vi "Controller.vi"(8 "Error In":errorcluster) -> (0 "Error Out":errorcluster)   [LabVIEW 2017]
uses:
  Controller Data Cluster.ctl
  User Console/UI Data Cluster.ctl
  Timed Action.ctl
  Current Direction.ctl
  Communication/Reference Action.ctl
  Display Console/Communication/Display Console Message.ctl
  Display Console/Display Console Data Cluster.ctl
  Communication/User Event/User Event Cluster.ctl
  Communication/User Event/User Event Enum.ctl
  Communication/Controller Queue Message.ctl
  Support VIs/Timer Actions.ctl
  Emergency Enum.ctl
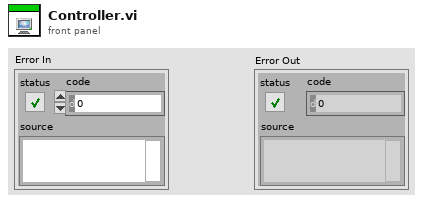
[diagram p1: front panel]
types:
  T1 = typedef "Controller Data Cluster.ctl" = cluster{"UI Data Cluster":T2, "Sensor Position":u32, "Module Closed?":cluster{"Display Loop":bool, "Sensor Loop ":bool}, "Time to Elapse":u32, "Request?":bool, "Timed Action":T3, "Time Constants":cluster{"Open Door":dbl, "Close Door":dbl, "Travel":dbl, "Inactivity":dbl}, "Inactivity":bool, "Current Floor":u32, "Current Direction":T4, "Travel?":bool, "Program Exit":bool[], "Emergency?":bool}
  T2 = typedef "UI Data Cluster.ctl" = cluster{"Floor Selection":bool[], "Elevator Call Up":bool[], "Elevator Call Down":bool[], "Door Buttons":cluster{"Open":bool, "Close":bool}, "Emergency":bool}
  T3 = typedef "Timed Action.ctl" = enum16{"Open Door", "Close Door", "Travel", "Inactivity"}
  T4 = typedef "Current Direction.ctl" = enum16{"Up", "Down", "Idle"}
  T5 = typedef "Reference Action.ctl" = enum16{"Set", "Get"}
  T6 = typedef "Controller Queue Message.ctl" = enum16{"Initialize", "User Console Update", "Sensor Update", "Wait for First Request", "Start and Move", "Analysis", "Continue Travel", "Stop at Floor", "Open and Close Door Sequence", "Close Door", "No Request Remaining", "Check Time", "Emergency Call", "Terminate Process", "Controller Exit", "Start Exit", "Error Handling"}
  T7 = typedef "Display Console Message.ctl" = enum16{"Update Location", "Initialize", "Update", "Update Time", "Update Emergency", "Errror Handling", "Exit"}
  T8 = typedef "Timer Actions.ctl" = enum16{"Reset", "Check Time"}
  T9 = typedef "Display Console Data Cluster.ctl" = cluster{"Timing":dbl, "Elevator Location":u32, "Elevator Direction":cluster{"Up":bool, "Down":bool}, "Door Open":bool, "Emergency":bool}
  T10 = typedef "User Event Enum.ctl" = enum16{"Update Controlls", "Disable Open/Close Controlls", "Disable Open Door Controll", "Enable Open/Close Controlls", "Disable All Controlls", "Controller Loop Closed"}
  T11 = typedef "Emergency Enum.ctl" = enum16{"Energency On", "Emergency Off", "Emergency Idle"}
  T12 = typedef "User Event Cluster.ctl" = cluster{"User Event Enum":T10, "UI Data Cluster":T2}
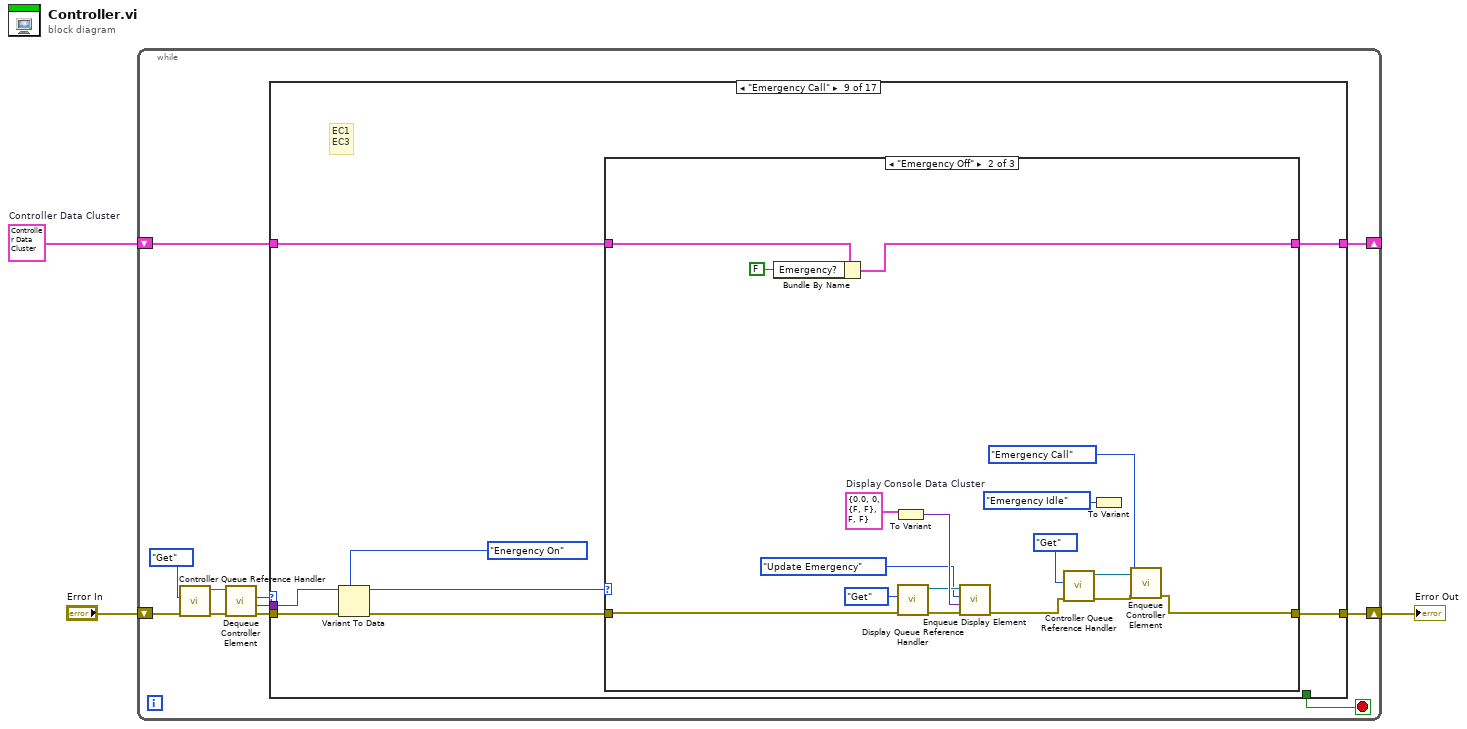
[diagram p0: block diagram]
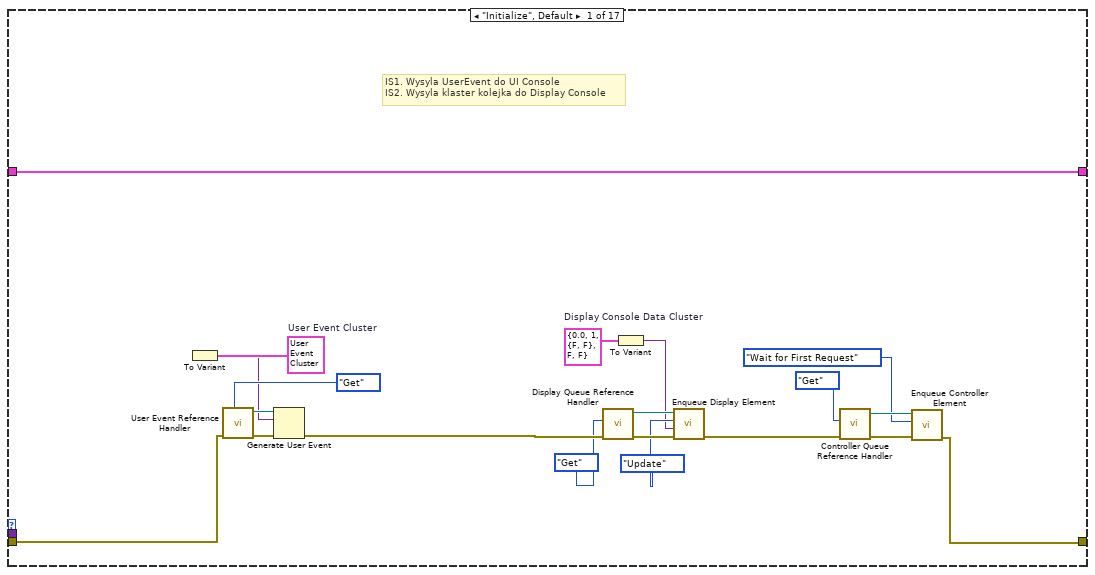
[diagram p2: hidden frame]
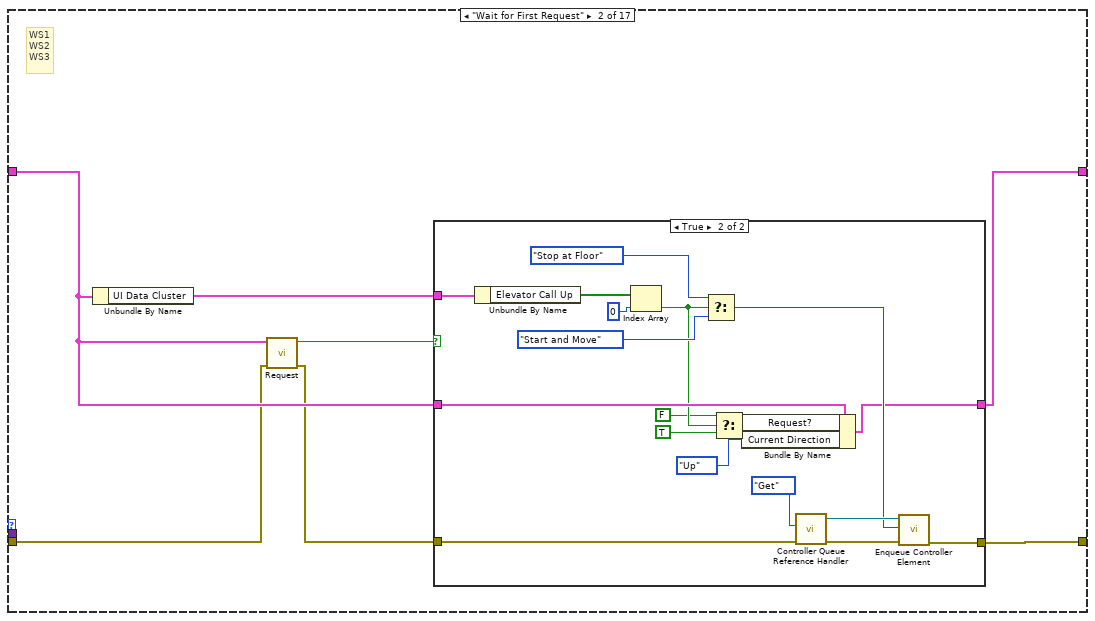
[diagram p3: hidden frame]
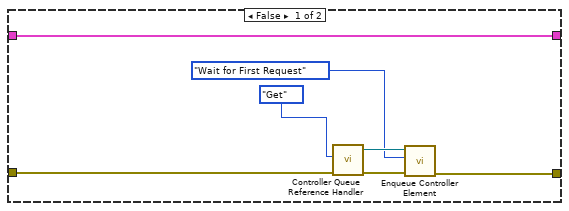
[diagram p4: hidden frame]
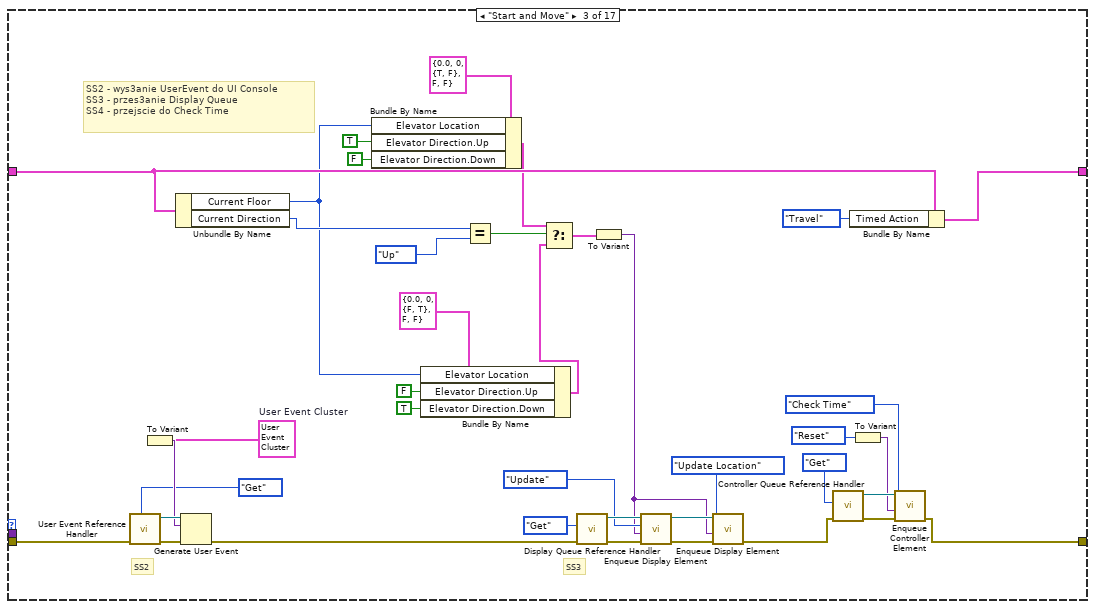
[diagram p5: hidden frame]
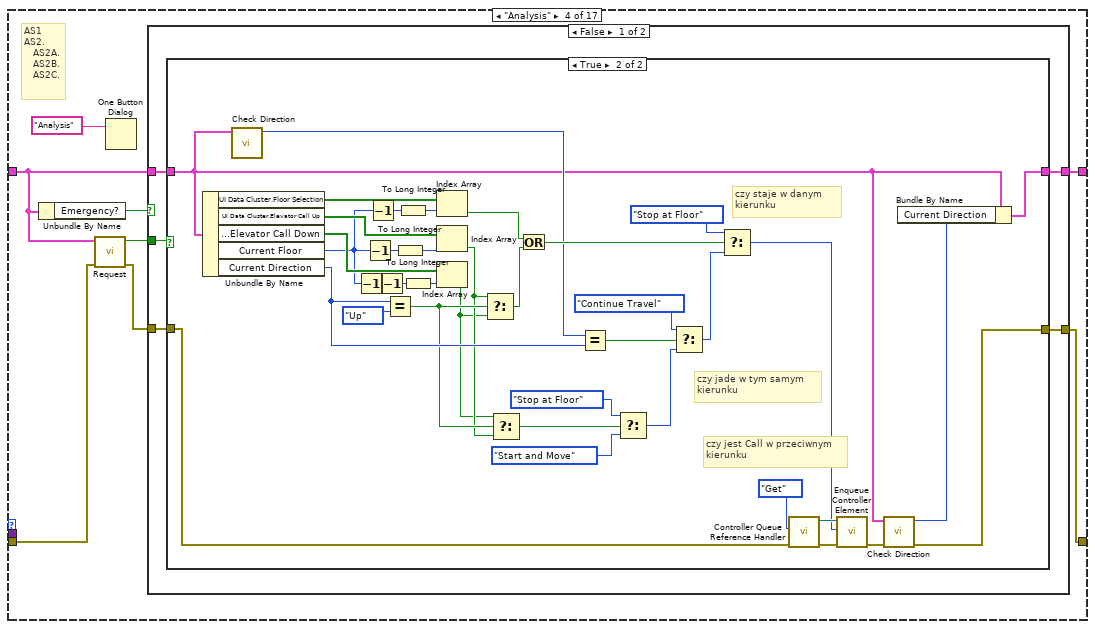
[diagram p6: hidden frame]
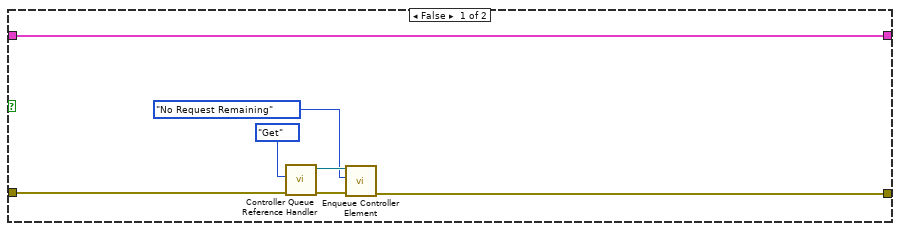
[diagram p7: hidden frame]
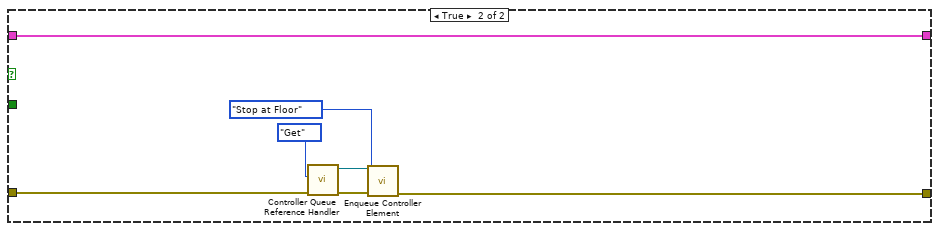
[diagram p8: hidden frame]
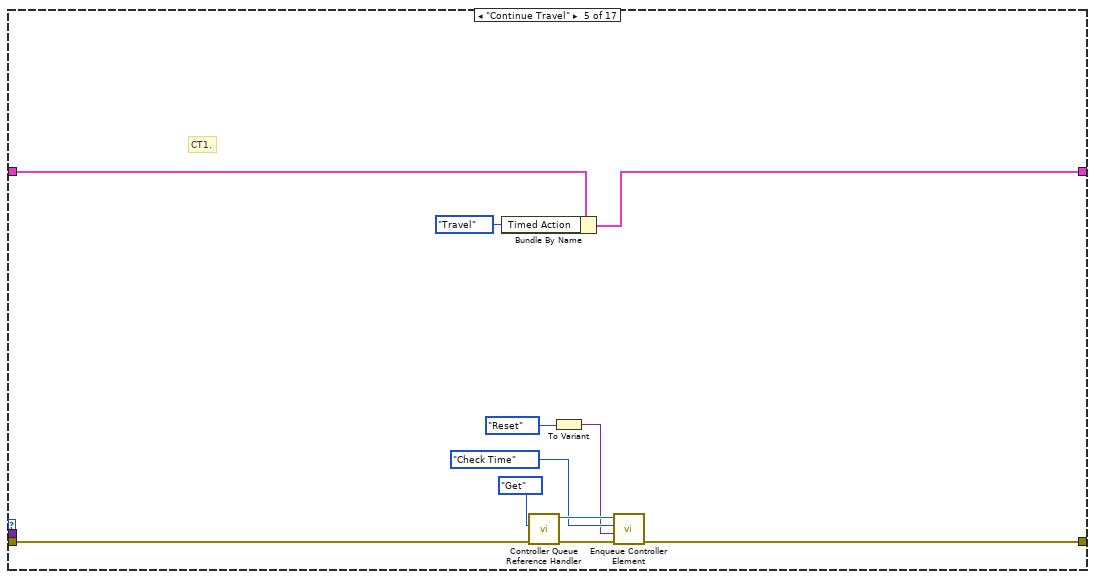
[diagram p9: hidden frame]
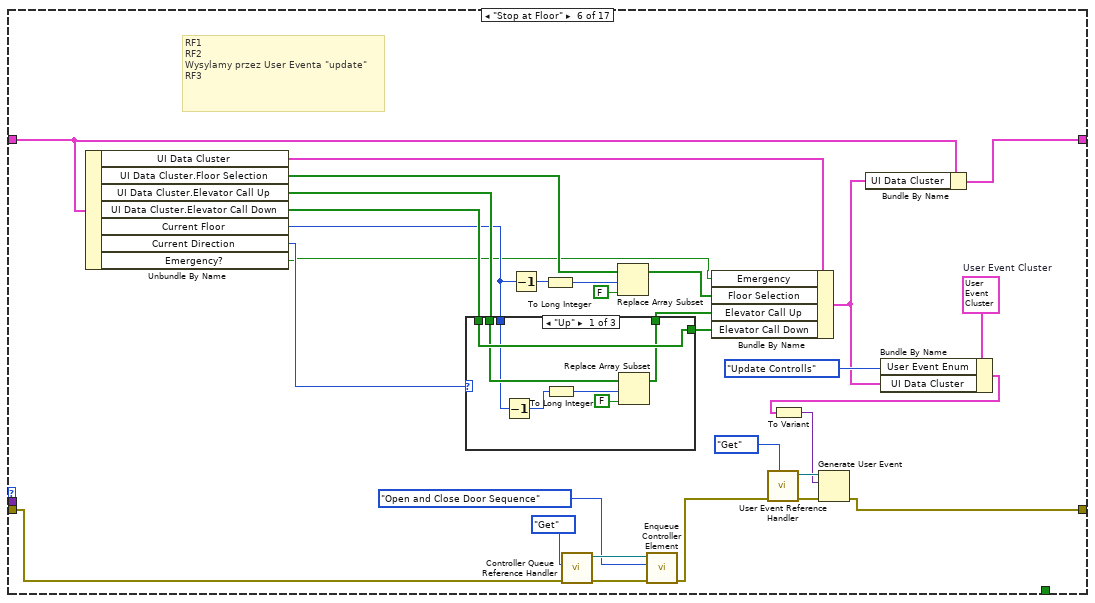
[diagram p10: hidden frame]
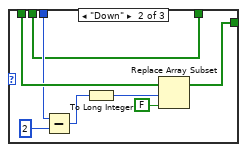
[diagram p11: hidden frame]
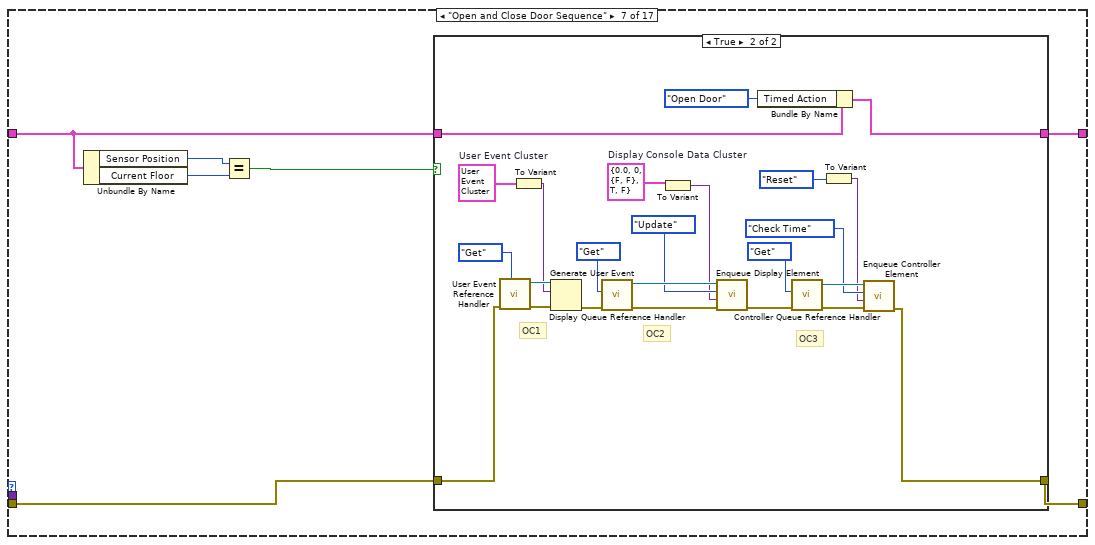
[diagram p13: hidden frame]
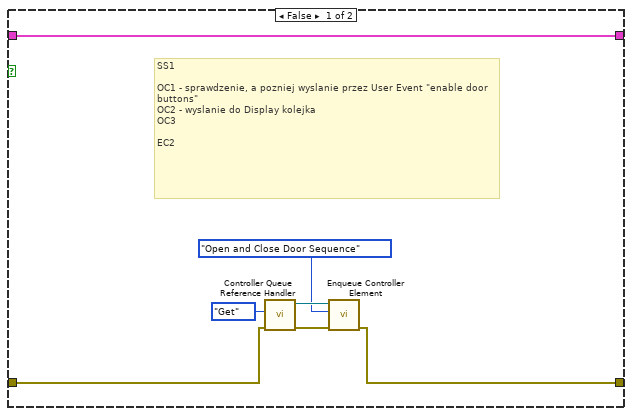
[diagram p14: hidden frame]
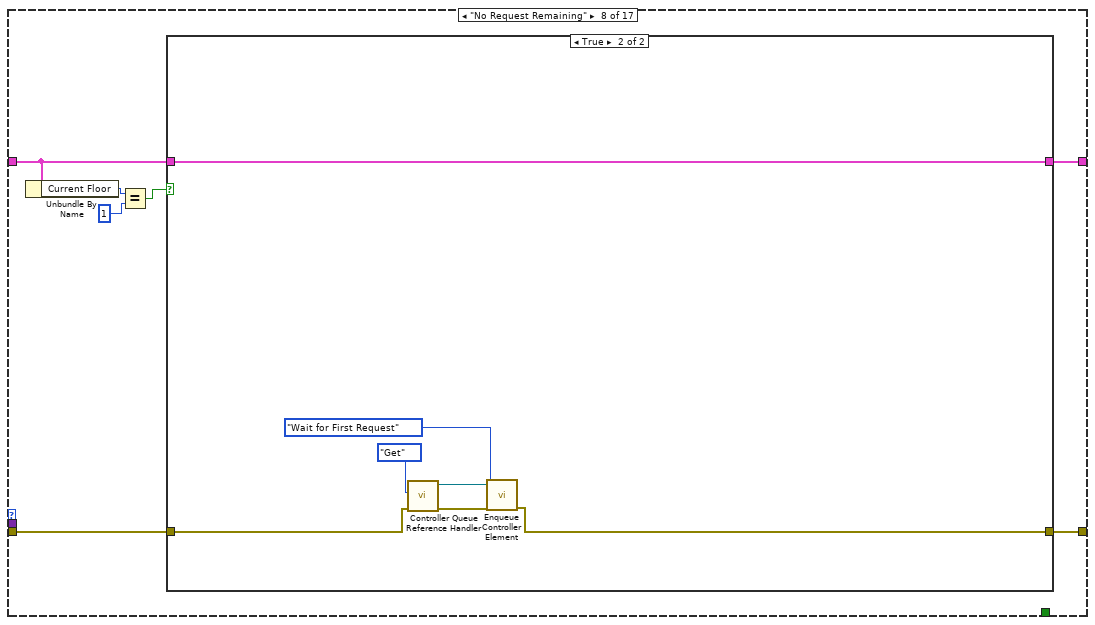
[diagram p15: hidden frame]
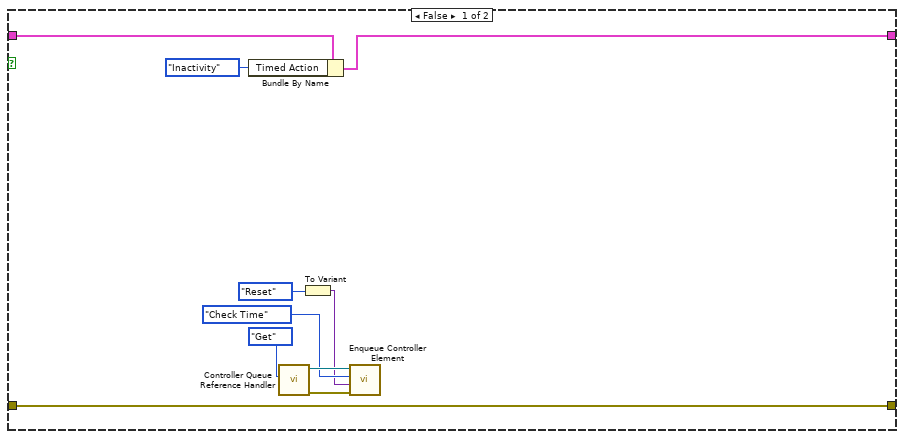
[diagram p16: hidden frame]
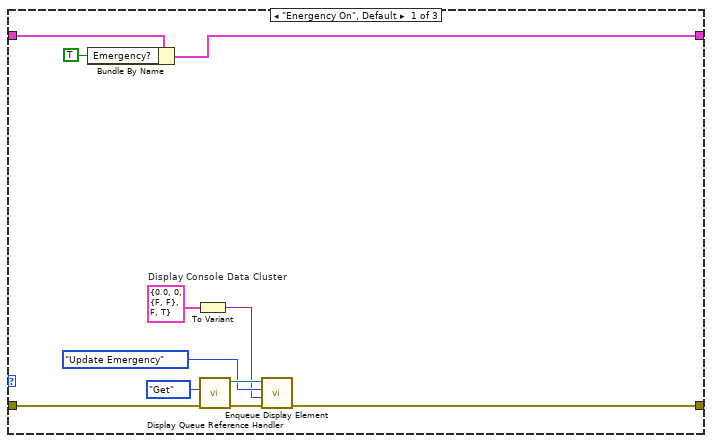
[diagram p17: hidden frame]
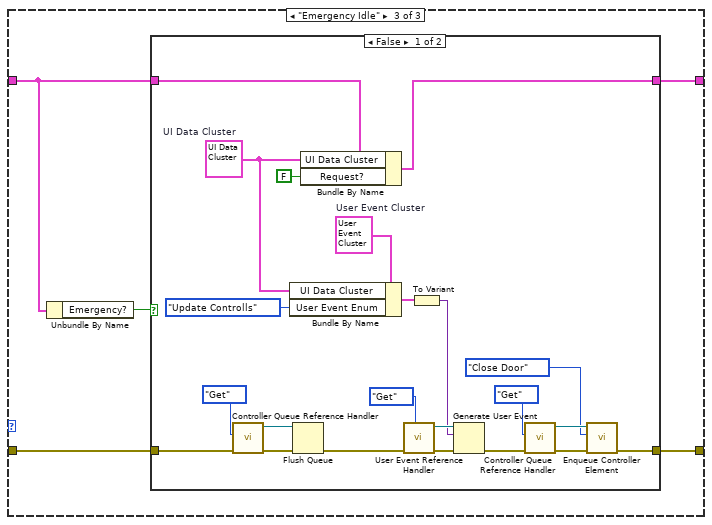
[diagram p18: hidden frame]
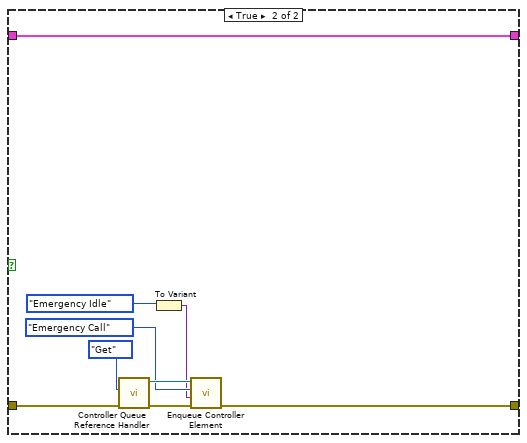
[diagram p19: hidden frame]
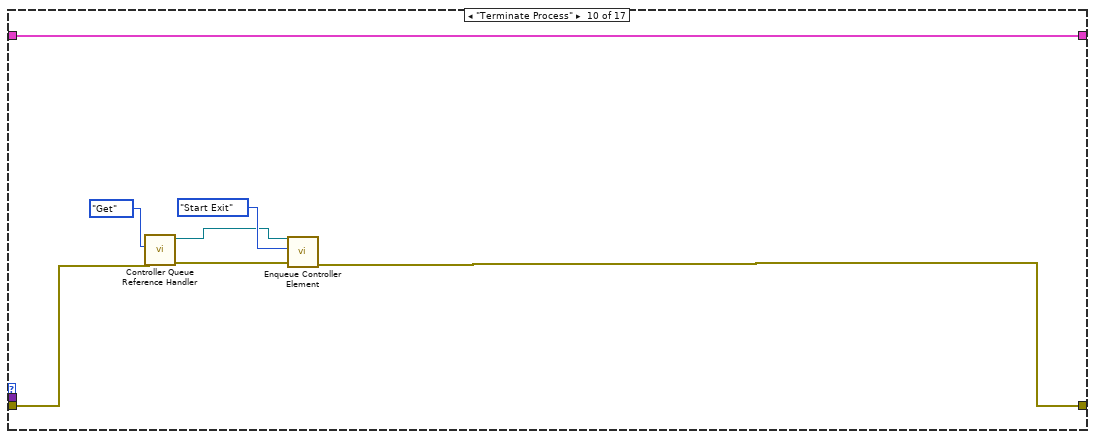
[diagram p20: hidden frame]
diagram:
  w1 = T1 {"UI Data Cluster"={"Floor Selection"=[], "Elevator Call Up"=[], "Elevator Call Down"=[], "Door Buttons"={"Open"=FALSE, "Close"=FALSE}, "Emergency"=FALSE}, "Sensor Position"=1, "Module Closed?"={"Display Loop"=FALSE, "Sensor Loop "=FALSE}, "Time to Elapse"=0, "Request?"=FALSE, "Timed Action"=enum."Open Door", "Time Constants"={"Open Door"=5.0, "Close Door"=1.0, "Travel"=10.0, "Inactivity"=20.0}, "Inactivity"=FALSE, "Current Floor"=1, "Current Direction"=enum."Idle", "Travel?"=FALSE, "Program Exit"=[], "Emergency?"=FALSE}  # Controller Data Cluster
  n1 = while {
    shift-right: [w12] -> w2
    shift-left: "Error In" -> [w14]
    shift-right: [w4] -> _
    shift-left: w1 -> [w7]
    stop <- w6 stop-if-true
    n2 = call "Controller Queue Reference Handler.vi"("Error In"=w14, "Reference Action"=Reference_Action."Get") -> ("Error Out"=w11:errorcluster, "Queue Ref Out"=w10:refnum<queue>)  [unwired: 8 in]
    n3 = call "Dequeue Controller Element.vi"("error in (no error)"=w11, "Message Queue"=w10) -> ("error out"=w8:errorcluster, "Controller Queue Data"=w5:variant, "Controller Queue Message"=w9:T6)  [unwired: 6 in, 1 out]
    n4 = case shown="\"Emergency Call\"" w9 {
      tunnel: w8 -> [w24 w37 w100 w107 w172 w185 w232 w269 w298 w365 w382 w388 w399 w405 w414 w659 w697]
      tunnel: [w15 w40 w84 w113 w171 w183 w231 w270 w293 w363 w381 w388 w398 w405 w408 w666 w678] -> w12
      tunnel: w7 -> [w32 w38 w89 w109 w180 w190 w230 w267 w291 w369 w371 w387 w392 w402 w410 w677 w693]
      tunnel: [w32 w39 w88 w112 w179 w195 w229 w268 w292 w369 w370 w387 w391 w401 w411 w677 w692] -> w4
      tunnel: [_ _ _ _ _ _ _ _ _ _ w374 _ _ _ _ _ _] -> w6
      tunnel: w5 -> [_ _ _ _ _ _ _ _ w297 _ w386 _ w400 w406 w415 _ _]
      frame "Initialize", Default {
        w22 = T12 {"User Event Enum"=enum."Update Controlls", "UI Data Cluster"={"Floor Selection"=[FALSE, FALSE, FALSE, FALSE], "Elevator Call Up"=[FALSE, FALSE, FALSE], "Elevator Call Down"=[FALSE, FALSE, FALSE], "Door Buttons"={"Open"=FALSE, "Close"=FALSE}, "Emergency"=FALSE}}  # User Event Cluster
        w25 = T9 {"Timing"=0.0, "Elevator Location"=1, "Elevator Direction"={"Up"=FALSE, "Down"=FALSE}, "Door Open"=FALSE, "Emergency"=FALSE}  # Display Console Data Cluster
        # "IS1. Wysyla UserEvent do UI Console \nIS2. Wysyla klaster kolejka do Display Console"
        n5 = To Variant(anything=w22) -> (Variant=w21:variant)
        n6 = call "User Event Reference Handler.vi"("Reference Action"=Reference_Action."Get", "Error In"=w24) -> ("Error Out"=w33:errorcluster, "User Event Refnum Out"=w34:refnum<user-event>)  [unwired: 7 in, 1 out]
        n7 = Generate User Event(user event=w34, event data cluster=w21, error in=w33) -> (error out=w29:errorcluster)  [unwired: 1 in, 1 out]
        n8 = call "Display Queue Reference Handler.vi"("Error In"=w29, "Reference Action"=Reference_Action."Get") -> ("Error Out"=w30:errorcluster, "Queue Ref Out"=w31:refnum<queue>)  [unwired: 8 in]
        n9 = To Variant(anything=w25) -> (Variant=w26:variant)
        n10 = call "Enqueue Display Element.vi"("error in (no error)"=w30, "Display Console Data"=w26, "Display Console Message"=Display_Console_Message."Update", "Message Queue"=w31) -> ("error out"=w16:errorcluster)  [unwired: 6 in, 1 out]
        n11 = call "Controller Queue Reference Handler.vi"("Error In"=w16, "Reference Action"=Reference_Action."Get") -> ("Error Out"=w19:errorcluster, "Queue Ref Out"=w18:refnum<queue>)  [unwired: 8 in]
        n12 = call "Enqueue Controller Element.vi"("error in (no error)"=w19, "Controller Queue Message"=Controller_Queue_Message."Wait for First Request", "Message Queue"=w18) -> ("error out"=w15:errorcluster)  [unwired: 7 in, 1 out]
      }
      frame "Wait for First Request" {
        # "WS1\nWS2\nWS3"
        n13 = Unbundle By Name(w38) -> ("UI Data Cluster"=w41:T2)
        n14 = call "Request.vi"("error in (no error)"=w37, "Controller Data Cluster"=w38) -> ("error out"=w36:errorcluster, "Request?"=w35:bool)  [unwired: 8 in]
        n15 = case shown="True" w35 {
          tunnel: w41 -> [_ w66]
          tunnel: w36 -> [w44 w57]
          tunnel: [w43 w56] -> w40
          tunnel: w38 -> [w42 w55]
          tunnel: [w42 w50] -> w39
          frame False {
            n16 = call "Controller Queue Reference Handler.vi"("Error In"=w44, "Reference Action"=Reference_Action."Get") -> ("Error Out"=w47:errorcluster, "Queue Ref Out"=w46:refnum<queue>)  [unwired: 8 in]
            n17 = call "Enqueue Controller Element.vi"("error in (no error)"=w47, "Controller Queue Message"=Controller_Queue_Message."Wait for First Request", "Message Queue"=w46) -> ("error out"=w43:errorcluster)  [unwired: 7 in, 1 out]
          }
          frame True {
            n18 = Unbundle By Name(w66) -> ("Elevator Call Up"=w65:bool[])
            n19 = Index Array(array=w65, index=0) -> (element=w53:bool)
            n20 = Select(t=Controller_Queue_Message."Stop at Floor" ("Controller Queue Message"), s=w53, f=Controller_Queue_Message."Start and Move" ("Controller Queue Message")) -> (s? t:f=w58:T6)
            n21 = Select(t=FALSE, s=w53, f=TRUE) -> (s? t:f=w54:bool)
            n22 = Bundle By Name(cluster=w55, "Request?"=w54, "Current Direction"=Current_Direction."Up") -> (w50:T1)
            n23 = call "Controller Queue Reference Handler.vi"("Error In"=w57, "Reference Action"=Reference_Action."Get") -> ("Error Out"=w62:errorcluster, "Queue Ref Out"=w61:refnum<queue>)  [unwired: 8 in]
            n24 = call "Enqueue Controller Element.vi"("error in (no error)"=w62, "Controller Queue Message"=w58, "Message Queue"=w61) -> ("error out"=w56:errorcluster)  [unwired: 7 in, 1 out]
          }
        }
      }
      frame "Start and Move" {
        w101 = T12 {"User Event Enum"=enum."Disable Open/Close Controlls", "UI Data Cluster"={"Floor Selection"=[], "Elevator Call Up"=[], "Elevator Call Down"=[], "Door Buttons"={"Open"=FALSE, "Close"=FALSE}, "Emergency"=FALSE}}  # User Event Cluster
        # "SS3"
        # "SS2"
        # "SS2 - wys3anie UserEvent do UI Console\nSS3 - przes3anie Display Queue\nSS4 - przejscie do Check Time"
        n25 = call "User Event Reference Handler.vi"("Reference Action"=Reference_Action."Get", "Error In"=w100) -> ("Error Out"=w103:errorcluster, "User Event Refnum Out"=w105:refnum<user-event>)  [unwired: 7 in, 1 out]
        n26 = To Variant(anything=w101) -> (Variant=w104:variant)
        n27 = Unbundle By Name(w89) -> ("Current Floor"=w76:u32, "Current Direction"=w99:T4)
        n28 = Generate User Event(user event=w105, event data cluster=w104, error in=w103) -> (error out=w91:errorcluster)  [unwired: 1 in, 1 out]
        n29 = Bundle By Name(cluster=T9 {"Timing"=0.0, "Elevator Location"=0, "Elevator Direction"={"Up"=TRUE, "Down"=FALSE}, "Door Open"=FALSE, "Emergency"=FALSE} ("Display Console Data Cluster"), "Elevator Location"=w76, "Elevator Direction.Up"=TRUE, "Elevator Direction.Down"=FALSE) -> (w78:T9)
        n30 = Bundle By Name(cluster=T9 {"Timing"=0.0, "Elevator Location"=0, "Elevator Direction"={"Up"=FALSE, "Down"=TRUE}, "Door Open"=FALSE, "Emergency"=FALSE} ("Display Console Data Cluster"), "Elevator Location"=w76, "Elevator Direction.Up"=FALSE, "Elevator Direction.Down"=TRUE) -> (w72:T9)
        n31 = Equal?(x=w99, y=Current_Direction."Up" ("Current Direction")) -> (x = y?=w97:bool)
        n32 = Select(t=w78, s=w97, f=w72) -> (s? t:f=w92:T9)
        n33 = call "Display Queue Reference Handler.vi"("Error In"=w91, "Reference Action"=Reference_Action."Get") -> ("Error Out"=w95:errorcluster, "Queue Ref Out"=w94:refnum<queue>)  [unwired: 8 in]
        n34 = To Variant(anything=w92) -> (Variant=w67:variant)
        n35 = call "Enqueue Display Element.vi"("error in (no error)"=w95, "Display Console Data"=w67, "Display Console Message"=Display_Console_Message."Update", "Message Queue"=w94) -> ("error out"=w71:errorcluster, "dup Message Queue"=w69:refnum<queue>)  [unwired: 6 in]
        n36 = call "Enqueue Display Element.vi"("error in (no error)"=w71, "Display Console Data"=w67, "Display Console Message"=Display_Console_Message."Update Location", "Message Queue"=w69) -> ("error out"=w70:errorcluster)  [unwired: 6 in, 1 out]
        n37 = call "Controller Queue Reference Handler.vi"("Error In"=w70, "Reference Action"=Reference_Action."Get") -> ("Error Out"=w86:errorcluster, "Queue Ref Out"=w85:refnum<queue>)  [unwired: 8 in]
        n38 = Bundle By Name(cluster=w89, "Timed Action"=Timed_Action."Travel") -> (w88:T1)
        n39 = To Variant(anything=Timer_Actions."Reset" ("TimerAction")) -> (Variant=w81:variant)
        n40 = call "Enqueue Controller Element.vi"("error in (no error)"=w86, "Controller Queue Data"=w81, "Controller Queue Message"=Controller_Queue_Message."Check Time", "Message Queue"=w85) -> ("error out"=w84:errorcluster)  [unwired: 6 in, 1 out]
      }
      frame "Analysis" {
        # "AS1\nAS2.\n   AS2A.\n   AS2B.\n   AS2C."
        n41 = Unbundle By Name(w109) -> ("Emergency?"=w110:bool)
        n42 = call "Request.vi"("error in (no error)"=w107, "Controller Data Cluster"=w109) -> ("error out"=w106:errorcluster, "Request?"=w108:bool)  [unwired: 8 in]
        n43 = One Button Dialog(message="Analysis") -> ()  [unwired: 1 in, 1 out]
        n44 = case shown="False" w110 {
          tunnel: w106 -> [w117 w167]
          tunnel: [w116 w166] -> w113
          tunnel: [w114 w164] -> w112
          tunnel: w109 -> [w115 w164]
          tunnel: w108 -> [w118 _]
          frame False {
            n45 = case shown="True" w118 {
              tunnel: w117 -> [w121 w130]
              tunnel: [w120 w126] -> w116
              tunnel: w115 -> [w119 w128]
              tunnel: [w119 w147] -> w114
              frame False {
                n46 = call "Controller Queue Reference Handler.vi"("Error In"=w121, "Reference Action"=Reference_Action."Get") -> ("Error Out"=w124:errorcluster, "Queue Ref Out"=w125:refnum<queue>)  [unwired: 8 in]
                n47 = call "Enqueue Controller Element.vi"("error in (no error)"=w124, "Controller Queue Message"=Controller_Queue_Message."No Request Remaining", "Message Queue"=w125) -> ("error out"=w120:errorcluster)  [unwired: 7 in, 1 out]
              }
              frame True {
                # "czy jest Call w przeciwnym\nkierunku"
                # "czy jade w tym samym \nkierunku"
                # "czy staje w danym kierunku"
                n48 = Unbundle By Name(w128) -> ("UI Data Cluster.Floor Selection"=w162:bool[], "UI Data Cluster.Elevator Call Up"=w159:bool[], "UI Data Cluster.Elevator Call Down"=w156:bool[], "Current Floor"=w155:u32, "Current Direction"=w145:T4)
                n49 = call "Check Direction.vi"("Controller Data Cluster"=w128) -> ("Direction"=w146:T4)  [unwired: 9 in, 1 out]
                n50 = Decrement(x=w155) -> (x-1=w154:u32)
                n51 = Decrement(x=w155) -> (x-1=w158:u32)
                n52 = Decrement(x=w155) -> (x-1=w161:u32)
                n53 = Decrement(x=w154) -> (x-1=w153:u32)
                n54 = Equal?(x=w145, y=Current_Direction."Up") -> (x = y?=w141:bool)
                n55 = To Long Integer(number=w158) -> (32bit integer=w157:i32)
                n56 = To Long Integer(number=w161) -> (32bit integer=w160:i32)
                n57 = To Long Integer(number=w153) -> (32bit integer=w152:i32)
                n58 = Index Array(array=w162, index=w160) -> (element=w151:bool)
                n59 = Index Array(array=w159, index=w157) -> (element=w140:bool)
                n60 = Index Array(array=w156, index=w152) -> (element=w139:bool)
                n61 = Select(t=w140, s=w141, f=w139) -> (s? t:f=w150:bool)
                n62 = Select(t=w139, s=w141, f=w140) -> (s? t:f=w138:bool)
                n63 = Or(x=w151, y=w150) -> (x .or. y?=w149:bool)
                n64 = Equal?(x=w146, y=w145) -> (x = y?=w144:bool)
                n65 = Select(t=Controller_Queue_Message."Stop at Floor" ("Controller Queue Message"), s=w138, f=Controller_Queue_Message."Start and Move") -> (s? t:f=w135:T6)
                n66 = Select(t=Controller_Queue_Message."Continue Travel" ("Controller Queue Message"), s=w144, f=w135) -> (s? t:f=w142:T6)
                n67 = Select(t=Controller_Queue_Message."Stop at Floor" ("Controller Queue Message"), s=w149, f=w142) -> (s? t:f=w131:T6)
                n68 = call "Controller Queue Reference Handler.vi"("Error In"=w130, "Reference Action"=Reference_Action."Get") -> ("Error Out"=w133:errorcluster, "Queue Ref Out"=w132:refnum<queue>)  [unwired: 8 in]
                n69 = call "Enqueue Controller Element.vi"("error in (no error)"=w133, "Controller Queue Message"=w131, "Message Queue"=w132) -> ("error out"=w129:errorcluster)  [unwired: 7 in, 1 out]
                n70 = call "Check Direction.vi"("error in (no error)"=w129, "Controller Data Cluster"=w128) -> ("error out"=w126:errorcluster, "Direction"=w127:T4)  [unwired: 8 in]
                n71 = Bundle By Name(cluster=w128, "Current Direction"=w127) -> (w147:T1)
              }
            }
          }
          frame True {
            n72 = call "Controller Queue Reference Handler.vi"("Error In"=w167, "Reference Action"=Reference_Action."Get") -> ("Error Out"=w169:errorcluster, "Queue Ref Out"=w168:refnum<queue>)  [unwired: 8 in]
            n73 = call "Enqueue Controller Element.vi"("error in (no error)"=w169, "Controller Queue Message"=Controller_Queue_Message."Stop at Floor", "Message Queue"=w168) -> ("error out"=w166:errorcluster)  [unwired: 7 in, 1 out]
          }
        }
      }
      frame "Continue Travel" {
        # "CT1."
        n74 = Bundle By Name(cluster=w180, "Timed Action"=Timed_Action."Travel") -> (w179:T1)
        n75 = call "Controller Queue Reference Handler.vi"("Error In"=w172, "Reference Action"=Reference_Action."Get") -> ("Error Out"=w177:errorcluster, "Queue Ref Out"=w176:refnum<queue>)  [unwired: 8 in]
        n76 = To Variant(anything=Timer_Actions."Reset" ("TimerAction")) -> (Variant=w173:variant)
        n77 = call "Enqueue Controller Element.vi"("error in (no error)"=w177, "Controller Queue Data"=w173, "Controller Queue Message"=Controller_Queue_Message."Check Time", "Message Queue"=w176) -> ("error out"=w171:errorcluster)  [unwired: 6 in, 1 out]
      }
      frame "Stop at Floor" {
        w193 = T12 {"User Event Enum"=enum."Update Controlls", "UI Data Cluster"={"Floor Selection"=[], "Elevator Call Up"=[], "Elevator Call Down"=[], "Door Buttons"={"Open"=FALSE, "Close"=FALSE}, "Emergency"=FALSE}}  # User Event Cluster
        # "RF1\nRF2\nWysylamy przez User Eventa \"update\"\nRF3"
        n78 = Unbundle By Name(w190) -> ("UI Data Cluster"=w196:T2, "UI Data Cluster.Floor Selection"=w206:bool[], "UI Data Cluster.Elevator Call Up"=w200:bool[], "UI Data Cluster.Elevator Call Down"=w201:bool[], "Current Floor"=w199:u32, "Current Direction"=w202:T4, "Emergency?"=w182:bool)
        n79 = case shown="\"Up\"" w202 {
          tunnel: w201 -> [w218 w224 w227]
          tunnel: w200 -> [w215 w219 w228]
          tunnel: w199 -> [w214 w223 _]
          tunnel: [w218 w220 w227] -> w198
          tunnel: [w212 w219 w228] -> w197
          frame "Up" {
            n80 = Decrement(x=w214) -> (x-1=w213:u32)
            n81 = To Long Integer(number=w213) -> (32bit integer=w217:i32)
            n82 = Replace Array Subset(array=w215, new element=FALSE ("new element/subarray"), index=w217) -> (w212:bool[])
          }
          frame "Down" {
            n83 = Subtract(x=w223, y=u32 2) -> (x-y=w221:u32)
            n84 = To Long Integer(number=w221) -> (32bit integer=w226:i32)
            n85 = Replace Array Subset(array=w224, new element=FALSE ("new element/subarray"), index=w226) -> (w220:bool[])
          }
          frame "Idle", Default {
          }
        }
        n86 = Decrement(x=w199) -> (x-1=w207:u32)
        n87 = To Long Integer(number=w207) -> (32bit integer=w205:i32)
        n88 = call "Controller Queue Reference Handler.vi"("Error In"=w185, "Reference Action"=Reference_Action."Get") -> ("Error Out"=w188:errorcluster, "Queue Ref Out"=w187:refnum<queue>)  [unwired: 8 in]
        n89 = Replace Array Subset(array=w206, new element=FALSE ("new element/subarray"), index=w205) -> (w203:bool[])
        n90 = call "Enqueue Controller Element.vi"("error in (no error)"=w188, "Controller Queue Message"=Controller_Queue_Message."Open and Close Door Sequence", "Message Queue"=w187) -> ("error out"=w184:errorcluster)  [unwired: 7 in, 1 out]
        n91 = Bundle By Name(cluster=w196, "Emergency"=w182, "Floor Selection"=w203, "Elevator Call Up"=w197, "Elevator Call Down"=w198) -> (w192:T2)
        n92 = call "User Event Reference Handler.vi"("Reference Action"=Reference_Action."Get", "Error In"=w184) -> ("Error Out"=w209:errorcluster, "User Event Refnum Out"=w211:refnum<user-event>)  [unwired: 7 in, 1 out]
        n93 = Bundle By Name(cluster=w190, "UI Data Cluster"=w192) -> (w195:T1)
        n94 = Bundle By Name(cluster=w193, "User Event Enum"=User_Event_Enum."Update Controlls", "UI Data Cluster"=w192) -> (w191:T12)
        n95 = To Variant(anything=w191) -> (Variant=w210:variant)
        n96 = Generate User Event(user event=w211, event data cluster=w210, error in=w209) -> (error out=w183:errorcluster)  [unwired: 1 in, 1 out]
      }
      frame "Open and Close Door Sequence" {
        n97 = Unbundle By Name(w230) -> ("Sensor Position"=w234:u32, "Current Floor"=w235:u32)
        n98 = Equal?(x=w234, y=w235) -> (x = y?=w233:bool)
        n99 = case shown="True" w233 {
          tunnel: w232 -> [w238 w248]
          tunnel: [w237 w247] -> w231
          tunnel: w230 -> [w236 w244]
          tunnel: [w236 w243] -> w229
          frame False {
            # "SS1\n\nOC1 - sprawdzenie, a pozniej wyslanie przez User Event \"enable door buttons\"\nOC2 - wyslanie do Display kolejka\nOC3\n\nEC2"
            n100 = call "Controller Queue Reference Handler.vi"("Error In"=w238, "Reference Action"=Reference_Action."Get") -> ("Error Out"=w241:errorcluster, "Queue Ref Out"=w240:refnum<queue>)  [unwired: 8 in]
            n101 = call "Enqueue Controller Element.vi"("error in (no error)"=w241, "Controller Queue Message"=Controller_Queue_Message."Open and Close Door Sequence", "Message Queue"=w240) -> ("error out"=w237:errorcluster)  [unwired: 7 in, 1 out]
          }
          frame True {
            w256 = T9 {"Timing"=0.0, "Elevator Location"=0, "Elevator Direction"={"Up"=FALSE, "Down"=FALSE}, "Door Open"=TRUE, "Emergency"=FALSE}  # Display Console Data Cluster
            w264 = T12 {"User Event Enum"=enum."Enable Open/Close Controlls", "UI Data Cluster"={"Floor Selection"=[], "Elevator Call Up"=[], "Elevator Call Down"=[], "Door Buttons"={"Open"=FALSE, "Close"=FALSE}, "Emergency"=FALSE}}  # User Event Cluster
            # "OC3"
            # "OC2"
            # "OC1"
            n102 = call "User Event Reference Handler.vi"("Reference Action"=Reference_Action."Get", "Error In"=w248) -> ("Error Out"=w265:errorcluster, "User Event Refnum Out"=w266:refnum<user-event>)  [unwired: 7 in, 1 out]
            n103 = To Variant(anything=w264) -> (Variant=w263:variant)
            n104 = Generate User Event(user event=w266, event data cluster=w263, error in=w265) -> (error out=w262:errorcluster)  [unwired: 1 in, 1 out]
            n105 = call "Display Queue Reference Handler.vi"("Error In"=w262, "Reference Action"=Reference_Action."Get") -> ("Error Out"=w261:errorcluster, "Queue Ref Out"=w260:refnum<queue>)  [unwired: 8 in]
            n106 = To Variant(anything=w256) -> (Variant=w255:variant)
            n107 = call "Enqueue Display Element.vi"("error in (no error)"=w261, "Display Console Data"=w255, "Display Console Message"=Display_Console_Message."Update", "Message Queue"=w260) -> ("error out"=w254:errorcluster)  [unwired: 6 in, 1 out]
            n108 = Bundle By Name(cluster=w244, "Timed Action"=Timed_Action."Open Door") -> (w243:T1)
            n109 = call "Controller Queue Reference Handler.vi"("Error In"=w254, "Reference Action"=Reference_Action."Get") -> ("Error Out"=w252:errorcluster, "Queue Ref Out"=w251:refnum<queue>)  [unwired: 8 in]
            n110 = To Variant(anything=Timer_Actions."Reset" ("TimerAction")) -> (Variant=w249:variant)
            n111 = call "Enqueue Controller Element.vi"("error in (no error)"=w252, "Controller Queue Data"=w249, "Controller Queue Message"=Controller_Queue_Message."Check Time", "Message Queue"=w251) -> ("error out"=w247:errorcluster)  [unwired: 6 in, 1 out]
          }
        }
      }
      frame "No Request Remaining" {
        n112 = Unbundle By Name(w267) -> ("Current Floor"=w272:u32)
        n113 = Equal?(x=w272, y=u32 1) -> (x = y?=w273:bool)
        n114 = case shown="True" w273 {
          tunnel: [w283 w286] -> w270
          tunnel: w269 -> [w283 w288]
          tunnel: [w275 w290] -> w268
          tunnel: w267 -> [w276 w290]
          frame False {
            n115 = Bundle By Name(cluster=w276, "Timed Action"=Timed_Action."Inactivity") -> (w275:T1)
            n116 = call "Controller Queue Reference Handler.vi"("Reference Action"=Reference_Action."Get") -> ("Error Out"=w281:errorcluster, "Queue Ref Out"=w280:refnum<queue>)  [unwired: 9 in]
            n117 = To Variant(anything=Timer_Actions."Reset" ("TimerAction")) -> (Variant=w277:variant)
            n118 = call "Enqueue Controller Element.vi"("error in (no error)"=w281, "Controller Queue Data"=w277, "Controller Queue Message"=Controller_Queue_Message."Check Time", "Message Queue"=w280) -> ()  [unwired: 6 in, 2 out]
          }
          frame True {
            n119 = call "Controller Queue Reference Handler.vi"("Error In"=w288, "Reference Action"=Reference_Action."Get") -> ("Error Out"=w287:errorcluster, "Queue Ref Out"=w285:refnum<queue>)  [unwired: 8 in]
            n120 = call "Enqueue Controller Element.vi"("error in (no error)"=w287, "Controller Queue Message"=Controller_Queue_Message."Wait for First Request", "Message Queue"=w285) -> ("error out"=w286:errorcluster)  [unwired: 7 in, 1 out]
          }
        }
      }
      frame "Emergency Call" {
        # "EC1\nEC3"
        n121 = Variant To Data(error in=w298, type=Emergency_Enum."Energency On" ("Emergency Enum"), Variant=w297) -> (data=w295:T11, error out=w294:errorcluster)
        n122 = case shown="\"Emergency Off\"" w295 {
          tunnel: w294 -> [w305 w317 w328]
          tunnel: [w304 w313 w329] -> w293
          tunnel: [w308 w325 w330] -> w292
          tunnel: w291 -> [w307 w326 w331]
          frame "Energency On", Default {
            w300 = T9 {"Timing"=0.0, "Elevator Location"=0, "Elevator Direction"={"Up"=FALSE, "Down"=FALSE}, "Door Open"=FALSE, "Emergency"=TRUE}  # Display Console Data Cluster
            n123 = Bundle By Name(cluster=w307, "Emergency?"=TRUE) -> (w308:T1)
            n124 = To Variant(anything=w300) -> (Variant=w299:variant)
            n125 = call "Display Queue Reference Handler.vi"("Error In"=w305, "Reference Action"=Reference_Action."Get") -> ("Error Out"=w306:errorcluster, "Queue Ref Out"=w302:refnum<queue>)  [unwired: 8 in]
            n126 = call "Enqueue Display Element.vi"("error in (no error)"=w306, "Display Console Data"=w299, "Display Console Message"=Display_Console_Message."Update Emergency", "Message Queue"=w302) -> ("error out"=w304:errorcluster)  [unwired: 6 in, 1 out]
          }
          frame "Emergency Off" {
            w318 = T9 {"Timing"=0.0, "Elevator Location"=0, "Elevator Direction"={"Up"=FALSE, "Down"=FALSE}, "Door Open"=FALSE, "Emergency"=FALSE}  # Display Console Data Cluster
            n127 = Bundle By Name(cluster=w326, "Emergency?"=FALSE) -> (w325:T1)
            n128 = To Variant(anything=w318) -> (Variant=w323:variant)
            n129 = call "Display Queue Reference Handler.vi"("Error In"=w317, "Reference Action"=Reference_Action."Get") -> ("Error Out"=w321:errorcluster, "Queue Ref Out"=w322:refnum<queue>)  [unwired: 8 in]
            n130 = call "Enqueue Display Element.vi"("error in (no error)"=w321, "Display Console Data"=w323, "Display Console Message"=Display_Console_Message."Update Emergency", "Message Queue"=w322) -> ("error out"=w316:errorcluster)  [unwired: 6 in, 1 out]
            n131 = call "Controller Queue Reference Handler.vi"("Error In"=w316, "Reference Action"=Reference_Action."Get") -> ("Error Out"=w314:errorcluster, "Queue Ref Out"=w312:refnum<queue>)  [unwired: 8 in]
            n132 = To Variant(anything=Emergency_Enum."Emergency Idle" ("Emergency Enum")) -> ()  [unwired: 1 out]
            n133 = call "Enqueue Controller Element.vi"("error in (no error)"=w314, "Controller Queue Message"=Controller_Queue_Message."Emergency Call", "Message Queue"=w312) -> ("error out"=w313:errorcluster)  [unwired: 7 in, 1 out]
          }
          frame "Emergency Idle" {
            n134 = Unbundle By Name(w331) -> ("Emergency?"=w327:bool)
            n135 = case shown="False" w327 {
              tunnel: w331 -> [w353 w362]
              tunnel: [w352 w362] -> w330
              tunnel: [w337 w358] -> w329
              tunnel: w328 -> [w335 w359]
              frame False {
                w347 = T12 {"User Event Enum"=enum."Update Controlls", "UI Data Cluster"={"Floor Selection"=[], "Elevator Call Up"=[], "Elevator Call Down"=[], "Door Buttons"={"Open"=FALSE, "Close"=FALSE}, "Emergency"=FALSE}}  # User Event Cluster
                w346 = T2 {"Floor Selection"=[FALSE, FALSE, FALSE, FALSE], "Elevator Call Up"=[FALSE, FALSE, FALSE], "Elevator Call Down"=[FALSE, FALSE, FALSE], "Door Buttons"={"Open"=FALSE, "Close"=FALSE}, "Emergency"=FALSE}  # UI Data Cluster
                n136 = call "Controller Queue Reference Handler.vi"("Error In"=w335, "Reference Action"=Reference_Action."Get") -> ("Error Out"=w333:errorcluster, "Queue Ref Out"=w334:refnum<queue>)  [unwired: 8 in]
                n137 = Bundle By Name(cluster=w347, "UI Data Cluster"=w346, "User Event Enum"=User_Event_Enum."Update Controlls") -> (w344:T12)
                n138 = Flush Queue(queue=w334, error in (no error)=w333) -> (error out=w332:errorcluster)  [unwired: 2 out]
                n139 = Bundle By Name(cluster=w353, "UI Data Cluster"=w346, "Request?"=FALSE) -> (w352:T1)
                n140 = call "User Event Reference Handler.vi"("Reference Action"=Reference_Action."Get", "Error In"=w332) -> ("Error Out"=w350:errorcluster, "User Event Refnum Out"=w349:refnum<user-event>)  [unwired: 7 in, 1 out]
                n141 = To Variant(anything=w344) -> (Variant=w343:variant)
                n142 = Generate User Event(user event=w349, event data cluster=w343, error in=w350) -> (error out=w338:errorcluster)  [unwired: 1 in, 1 out]
                n143 = call "Controller Queue Reference Handler.vi"("Error In"=w338, "Reference Action"=Reference_Action."Get") -> ("Error Out"=w341:errorcluster, "Queue Ref Out"=w340:refnum<queue>)  [unwired: 8 in]
                n144 = call "Enqueue Controller Element.vi"("error in (no error)"=w341, "Controller Queue Message"=Controller_Queue_Message."Close Door", "Message Queue"=w340) -> ("error out"=w337:errorcluster)  [unwired: 7 in, 1 out]
              }
              frame True {
                n145 = call "Controller Queue Reference Handler.vi"("Error In"=w359, "Reference Action"=Reference_Action."Get") -> ("Error Out"=w360:errorcluster, "Queue Ref Out"=w357:refnum<queue>)  [unwired: 8 in]
                n146 = To Variant(anything=Emergency_Enum."Emergency Idle" ("Emergency Enum")) -> (Variant=w354:variant)
                n147 = call "Enqueue Controller Element.vi"("error in (no error)"=w360, "Controller Queue Data"=w354, "Controller Queue Message"=Controller_Queue_Message."Emergency Call", "Message Queue"=w357) -> ("error out"=w358:errorcluster)  [unwired: 6 in, 1 out]
              }
            }
          }
        }
      }
      frame "Terminate Process" {
        n148 = call "Controller Queue Reference Handler.vi"("Error In"=w365, "Reference Action"=Reference_Action."Get") -> ("Error Out"=w364:errorcluster, "Queue Ref Out"=w366:refnum<queue>)  [unwired: 8 in]
        n149 = call "Enqueue Controller Element.vi"("error in (no error)"=w364, "Controller Queue Message"=Controller_Queue_Message."Start Exit", "Message Queue"=w366) -> ("error out"=w363:errorcluster)  [unwired: 7 in, 1 out]
      }
      frame "Controller Exit" {
        # "TS1 - wyslanie User Eventa\nTS2\nTS3, TS4 - wyslanie do Display kolejka"
        n150 = Unbundle By Name(w371) -> ("Program Exit"=w373:bool[])
        n151 = Variant To Data(error in=w382, type=0, Variant=w386) -> (data=w384:i32, error out=w381:errorcluster)
        n152 = Insert Into Array(array=w373, index=w384, new element=TRUE) -> (w372:bool[])
        n153 = Index Array(array=w372, index=0) -> (element=w377:bool)
        n154 = Index Array(array=w372, index=1) -> (element=w376:bool)
        n155 = Index Array(array=w372, index=2) -> (element=w375:bool)
        n156 = Bundle By Name(cluster=w371, "Program Exit"=w372) -> (w370:T1)
        n157 = Compound Arithmetic op=AND(w377, w376, w375) -> (w374:bool)
      }
      frame "Error Handling" {
        # "EH1-EH4"
      }
      frame "User Console Update" {
        w390 = T1 {"UI Data Cluster"={"Floor Selection"=[], "Elevator Call Up"=[], "Elevator Call Down"=[], "Door Buttons"={"Open"=FALSE, "Close"=FALSE}, "Emergency"=FALSE}, "Sensor Position"=0, "Module Closed?"={"Display Loop"=FALSE, "Sensor Loop "=FALSE}, "Time to Elapse"=0, "Request?"=FALSE, "Timed Action"=enum."Open Door", "Time Constants"={"Open Door"=0.0, "Close Door"=0.0, "Travel"=0.0, "Inactivity"=0.0}, "Inactivity"=FALSE, "Current Floor"=0, "Current Direction"=enum."Up", "Travel?"=FALSE, "Program Exit"=[], "Emergency?"=FALSE}  # Controller Data Cluster
        n158 = Variant To Data(error in=w399, type=w390, Variant=w400) -> (data=w397:T1, error out=w398:errorcluster)
        n159 = Unbundle By Name(w397) -> ("UI Data Cluster.Floor Selection"=w396:bool[], "UI Data Cluster.Elevator Call Up"=w395:bool[], "UI Data Cluster.Elevator Call Down"=w394:bool[], "Request?"=w389:bool)
        n160 = One Button Dialog(message="Naciśnięto przycisk na User Console") -> ()  [unwired: 1 in, 1 out]
        n161 = Bundle By Name(cluster=w392, "UI Data Cluster.Floor Selection"=w396, "UI Data Cluster.Elevator Call Up"=w395, "UI Data Cluster.Elevator Call Down"=w394, "Request?"=w389) -> (w391:T1)
      }
      frame "Sensor Update" {
        n162 = Variant To Data(error in=w405, type=u32 0, Variant=w406) -> (data=w403:u32)  [unwired: 1 out]
        n163 = Bundle By Name(cluster=w402, "Sensor Position"=w403) -> (w401:T1)
      }
      frame "Check Time" {
        n164 = Unbundle By Name(w410) -> ("Timed Action"=w409:T3)
        n165 = Variant To Data(error in=w414, type=Timer_Actions."Reset" ("TimerAction"), Variant=w415) -> (data=w412:T8, error out=w407:errorcluster)
        n166 = case shown="\"Open Door\", Default" w409 {
          tunnel: w412 -> [w423 w464 w518 w608]
          tunnel: [w418 w459 w513 w603] -> w411
          tunnel: w410 -> [w417 w458 w512 w602]
          tunnel: [w421 w462 w516 w606] -> w408
          tunnel: w407 -> [w424 w465 w519 w609]
          frame "Open Door", Default {
            n167 = Unbundle By Name(w417) -> ("Time Constants.Open Door"=w416:dbl)
            n168 = call "Timer.vi"("TimerAction"=w423, "error in (no error)"=w424, "Time To Elapse"=w416) -> ("error out"=w422:errorcluster, "TimeElapsed?"=w420:bool, "Elapsed Time"=w419:dbl)  [unwired: 6 in]
            n169 = case shown="False" w420 {
              tunnel: w422 -> [w443 w453]
              tunnel: [w428 w452] -> w421
              tunnel: w419 -> [w427 _]
              tunnel: [w444 w451] -> w418
              tunnel: w417 -> [w444 w451]
              tunnel: w416 -> [w426 _]
              frame False {
                w441 = T9 {"Timing"=0.0, "Elevator Location"=0, "Elevator Direction"={"Up"=FALSE, "Down"=FALSE}, "Door Open"=FALSE, "Emergency"=FALSE}  # Display Console Data Cluster
                n170 = Subtract(x=w426, y=w427) -> (x-y=w425:dbl)
                n171 = Bundle By Name(cluster=w441, "Timing"=w425) -> (w440:T9)
                n172 = call "Display Queue Reference Handler.vi"("Error In"=w443, "Reference Action"=Reference_Action."Get") -> ("Error Out"=w442:errorcluster, "Queue Ref Out"=w438:refnum<queue>)  [unwired: 8 in]
                n173 = To Variant(anything=w440) -> (Variant=w439:variant)
                n174 = call "Enqueue Display Element.vi"("error in (no error)"=w442, "Display Console Data"=w439, "Display Console Message"=Display_Console_Message."Update Time", "Message Queue"=w438) -> ("error out"=w435:errorcluster)  [unwired: 6 in, 1 out]
                n175 = call "Controller Queue Reference Handler.vi"("Error In"=w435, "Reference Action"=Reference_Action."Get") -> ("Error Out"=w433:errorcluster, "Queue Ref Out"=w432:refnum<queue>)  [unwired: 8 in]
                n176 = To Variant(anything=Timer_Actions."Check Time" ("TimerAction")) -> (Variant=w429:variant)
                n177 = call "Enqueue Controller Element.vi"("error in (no error)"=w433, "Controller Queue Data"=w429, "Controller Queue Message"=Controller_Queue_Message."Check Time", "Message Queue"=w432) -> ("error out"=w428:errorcluster)  [unwired: 6 in, 1 out]
              }
              frame True {
                n178 = Unbundle By Name(w451) -> ("Emergency?"=w448:bool)
                n179 = To Variant(anything=Emergency_Enum."Emergency Idle" ("Emergency Enum")) -> (Variant=w449:variant)
                n180 = call "Controller Queue Reference Handler.vi"("Error In"=w453, "Reference Action"=Reference_Action."Get") -> ("Error Out"=w455:errorcluster, "Queue Ref Out"=w454:refnum<queue>)  [unwired: 8 in]
                n181 = Select(t=Controller_Queue_Message."Emergency Call" ("Controller Queue Message"), s=w448, f=Controller_Queue_Message."Close Door" ("Controller Queue Message")) -> (s? t:f=w445:T6)
                n182 = call "Enqueue Controller Element.vi"("error in (no error)"=w455, "Controller Queue Data"=w449, "Controller Queue Message"=w445, "Message Queue"=w454) -> ("error out"=w452:errorcluster)  [unwired: 6 in, 1 out]
              }
            }
          }
          frame "Inactivity" {
            n183 = Unbundle By Name(w458) -> ("Time Constants.Inactivity"=w457:dbl)
            n184 = call "Timer.vi"("TimerAction"=w464, "error in (no error)"=w465, "Time To Elapse"=w457) -> ("error out"=w463:errorcluster, "TimeElapsed?"=w461:bool, "Elapsed Time"=w460:dbl)  [unwired: 6 in]
            n185 = case shown="False" w461 {
              tunnel: w463 -> [w467 w507]
              tunnel: [w472 w506] -> w462
              tunnel: w460 -> [w471 _]
              tunnel: [w469 w500] -> w459
              tunnel: w458 -> [w469 w501]
              tunnel: w457 -> [w470 _]
              frame False {
                n186 = call "Request.vi"("error in (no error)"=w467, "Controller Data Cluster"=w469) -> ("error out"=w466:errorcluster, "Request?"=w468:bool)  [unwired: 8 in]
                n187 = case shown="True" w468 {
                  tunnel: w466 -> [w491 w496]
                  tunnel: [w476 w493] -> w472
                  tunnel: w471 -> [w475 _]
                  tunnel: w470 -> [w474 _]
                  frame False {
                    w489 = T9 {"Timing"=0.0, "Elevator Location"=0, "Elevator Direction"={"Up"=FALSE, "Down"=FALSE}, "Door Open"=FALSE, "Emergency"=FALSE}  # Display Console Data Cluster
                    n188 = Subtract(x=w474, y=w475) -> (x-y=w473:dbl)
                    n189 = Bundle By Name(cluster=w489, "Timing"=w473) -> (w488:T9)
                    n190 = call "Display Queue Reference Handler.vi"("Error In"=w491, "Reference Action"=Reference_Action."Get") -> ("Error Out"=w490:errorcluster, "Queue Ref Out"=w486:refnum<queue>)  [unwired: 8 in]
                    n191 = To Variant(anything=w488) -> (Variant=w487:variant)
                    n192 = call "Enqueue Display Element.vi"("error in (no error)"=w490, "Display Console Data"=w487, "Display Console Message"=Display_Console_Message."Update Time", "Message Queue"=w486) -> ("error out"=w483:errorcluster)  [unwired: 6 in, 1 out]
                    n193 = call "Controller Queue Reference Handler.vi"("Error In"=w483, "Reference Action"=Reference_Action."Get") -> ("Error Out"=w481:errorcluster, "Queue Ref Out"=w480:refnum<queue>)  [unwired: 8 in]
                    n194 = To Variant(anything=Timer_Actions."Check Time" ("TimerAction")) -> (Variant=w477:variant)
                    n195 = call "Enqueue Controller Element.vi"("error in (no error)"=w481, "Controller Queue Data"=w477, "Controller Queue Message"=Controller_Queue_Message."Check Time", "Message Queue"=w480) -> ("error out"=w476:errorcluster)  [unwired: 6 in, 1 out]
                  }
                  frame True {
                    n196 = call "Controller Queue Reference Handler.vi"("Error In"=w496, "Reference Action"=Reference_Action."Get") -> ("Error Out"=w495:errorcluster, "Queue Ref Out"=w494:refnum<queue>)  [unwired: 8 in]
                    n197 = call "Enqueue Controller Element.vi"("error in (no error)"=w495, "Controller Queue Message"=Controller_Queue_Message."Analysis", "Message Queue"=w494) -> ("error out"=w493:errorcluster)  [unwired: 7 in, 1 out]
                  }
                }
              }
              frame True {
                n198 = Unbundle By Name(w501) -> ("UI Data Cluster.Floor Selection"=w505:bool[])
                n199 = Insert Into Array(array=w505, index=0, new element=TRUE ("new element/subarray")) -> (w502:bool[])
                n200 = Bundle By Name(cluster=w501, "UI Data Cluster.Floor Selection"=w502, "Current Direction"=Current_Direction."Down") -> (w500:T1)
                n201 = call "Controller Queue Reference Handler.vi"("Error In"=w507, "Reference Action"=Reference_Action."Get") -> ("Error Out"=w509:errorcluster, "Queue Ref Out"=w508:refnum<queue>)  [unwired: 8 in]
                n202 = call "Enqueue Controller Element.vi"("error in (no error)"=w509, "Controller Queue Message"=Controller_Queue_Message."Start and Move", "Message Queue"=w508) -> ("error out"=w506:errorcluster)  [unwired: 7 in, 1 out]
              }
            }
          }
          frame "Travel" {
            n203 = Unbundle By Name(w512) -> ("Time Constants.Travel"=w511:dbl)
            n204 = call "Timer.vi"("TimerAction"=w518, "error in (no error)"=w519, "Time To Elapse"=w511) -> ("error out"=w517:errorcluster, "TimeElapsed?"=w515:bool, "Elapsed Time"=w514:dbl)  [unwired: 6 in]
            n205 = case shown="True" w515 {
              tunnel: w517 -> [w541 w557]
              tunnel: [w526 w555] -> w516
              tunnel: w514 -> [w525 _]
              tunnel: [w520 w556] -> w513
              tunnel: w512 -> [w521 w554]
              tunnel: w511 -> [w524 _]
              frame False {
                w539 = T9 {"Timing"=0.0, "Elevator Location"=0, "Elevator Direction"={"Up"=FALSE, "Down"=FALSE}, "Door Open"=FALSE, "Emergency"=FALSE}  # Display Console Data Cluster
                n206 = Subtract(x=w524, y=w525) -> (x-y=w523:dbl)
                n207 = Bundle By Name(cluster=w539, "Timing"=w523) -> (w538:T9)
                n208 = call "Display Queue Reference Handler.vi"("Error In"=w541, "Reference Action"=Reference_Action."Get") -> ("Error Out"=w540:errorcluster, "Queue Ref Out"=w536:refnum<queue>)  [unwired: 8 in]
                n209 = To Variant(anything=w538) -> (Variant=w537:variant)
                n210 = call "Enqueue Display Element.vi"("error in (no error)"=w540, "Display Console Data"=w537, "Display Console Message"=Display_Console_Message."Update Time", "Message Queue"=w536) -> ("error out"=w533:errorcluster)  [unwired: 6 in, 1 out]
                n211 = Bundle By Name(cluster=w521, "Travel?"=TRUE) -> (w520:T1)
                n212 = call "Controller Queue Reference Handler.vi"("Error In"=w533, "Reference Action"=Reference_Action."Get") -> ("Error Out"=w531:errorcluster, "Queue Ref Out"=w530:refnum<queue>)  [unwired: 8 in]
                n213 = To Variant(anything=Timer_Actions."Check Time" ("TimerAction")) -> (Variant=w527:variant)
                n214 = call "Enqueue Controller Element.vi"("error in (no error)"=w531, "Controller Queue Data"=w527, "Controller Queue Message"=Controller_Queue_Message."Check Time", "Message Queue"=w530) -> ("error out"=w526:errorcluster)  [unwired: 6 in, 1 out]
              }
              frame True {
                n215 = Unbundle By Name(w554) -> ("Sensor Position"=w544:u32, "Current Floor"=w546:u32, "Current Direction"=w545:T4)
                n216 = Equal?(x=w545, y=Current_Direction."Up" ("Current Direction")) -> (x = y?=w553:bool)
                n217 = To Long Integer(number=w546) -> (32bit integer=w551:i32)
                n218 = Select(t=1, s=w553, f=-1) -> (s? t:f=w550:i32)
                n219 = Add(x=w551, y=w550) -> (x+y=w552:i32)
                n220 = To Unsigned Long Integer(number=w552) -> (unsigned 32bit integer=w543:u32)
                n221 = Equal?(x=w544, y=w543) -> (x = y?=w542:bool)
                n222 = case shown="True" w542 {
                  tunnel: w557 -> [w559 w596]
                  tunnel: w554 -> [w566 w587]
                  tunnel: [w566 w586] -> w556
                  tunnel: [w558 w574] -> w555
                  frame False {
                    n223 = call "Controller Queue Reference Handler.vi"("Error In"=w559, "Reference Action"=Reference_Action."Get") -> ("Error Out"=w564:errorcluster, "Queue Ref Out"=w563:refnum<queue>)  [unwired: 8 in]
                    n224 = To Variant(anything=Timer_Actions."Check Time" ("TimerAction")) -> (Variant=w560:variant)
                    n225 = call "Enqueue Controller Element.vi"("error in (no error)"=w564, "Controller Queue Data"=w560, "Controller Queue Message"=Controller_Queue_Message."Check Time", "Message Queue"=w563) -> ("error out"=w558:errorcluster)  [unwired: 6 in, 1 out]
                  }
                  frame True {
                    n226 = Unbundle By Name(w587) -> ("Current Floor"=w591:u32, "Current Direction"=w595:T4)
                    n227 = call "Controller Queue Reference Handler.vi"("Error In"=w596, "Reference Action"=Reference_Action."Get") -> ("Error Out"=w599:errorcluster, "Queue Ref Out"=w598:refnum<queue>)  [unwired: 8 in]
                    n228 = call "Enqueue Controller Element.vi"("error in (no error)"=w599, "Controller Queue Message"=Controller_Queue_Message."Analysis", "Message Queue"=w598) -> ("error out"=w575:errorcluster)  [unwired: 7 in, 1 out]
                    n229 = Equal?(x=w595, y=Current_Direction."Up" ("Current Direction")) -> (x = y?=w581:bool)
                    n230 = call "Display Queue Reference Handler.vi"("Error In"=w575, "Reference Action"=Reference_Action."Get") -> ("Error Out"=w572:errorcluster, "Queue Ref Out"=w569:refnum<queue>)  [unwired: 8 in]
                    n231 = To Long Integer(number=w591) -> (32bit integer=w589:i32)
                    n232 = Select(t=1, s=w581, f=-1) -> (s? t:f=w590:i32)
                    n233 = Add(x=w589, y=w590) -> (x+y=w588:i32)
                    n234 = Select(t=TRUE, s=w581, f=FALSE) -> (s? t:f=w578:bool)
                    n235 = To Unsigned Long Integer(number=w588) -> (unsigned 32bit integer=w582:u32)
                    n236 = Not(x=w578) -> (.not. x?=w577:bool)
                    n237 = Bundle By Name(cluster=T9 {"Timing"=0.0, "Elevator Location"=0, "Elevator Direction"={"Up"=FALSE, "Down"=FALSE}, "Door Open"=FALSE, "Emergency"=FALSE} ("Display Console Data Cluster"), "Elevator Location"=w582, "Elevator Direction.Up"=w578, "Elevator Direction.Down"=w577) -> (w576:T9)
                    n238 = Bundle By Name(cluster=w587, "Current Floor"=w582, "Travel?"=FALSE) -> (w586:T1)
                    n239 = To Variant(anything=w576) -> (Variant=w567:variant)
                    n240 = call "Enqueue Display Element.vi"("error in (no error)"=w572, "Display Console Data"=w567, "Display Console Message"=Display_Console_Message."Update Location", "Message Queue"=w569) -> ("error out"=w571:errorcluster, "dup Message Queue"=w570:refnum<queue>)  [unwired: 6 in]
                    n241 = call "Enqueue Display Element.vi"("error in (no error)"=w571, "Display Console Data"=w567, "Display Console Message"=Display_Console_Message."Update", "Message Queue"=w570) -> ("error out"=w574:errorcluster)  [unwired: 6 in, 1 out]
                  }
                }
              }
            }
          }
          frame "Close Door" {
            n242 = Unbundle By Name(w602) -> ("Time Constants.Close Door"=w601:dbl)
            n243 = call "Timer.vi"("TimerAction"=w608, "error in (no error)"=w609, "Time To Elapse"=w601) -> ("error out"=w607:errorcluster, "TimeElapsed?"=w605:bool, "Elapsed Time"=w604:dbl)  [unwired: 6 in]
            n244 = case shown="False" w605 {
              tunnel: w607 -> [w628 w634]
              tunnel: [w613 w637] -> w606
              tunnel: w604 -> [w612 _]
              tunnel: [w629 w630] -> w603
              tunnel: w602 -> [w629 w631]
              tunnel: w601 -> [w611 _]
              frame False {
                w626 = T9 {"Timing"=0.0, "Elevator Location"=0, "Elevator Direction"={"Up"=FALSE, "Down"=FALSE}, "Door Open"=FALSE, "Emergency"=FALSE}  # Display Console Data Cluster
                # "OC5"
                n245 = Subtract(x=w611, y=w612) -> (x-y=w610:dbl)
                n246 = Bundle By Name(cluster=w626, "Timing"=w610) -> (w625:T9)
                n247 = To Variant(anything=w625) -> (Variant=w624:variant)
                n248 = call "Display Queue Reference Handler.vi"("Error In"=w628, "Reference Action"=Reference_Action."Get") -> ("Error Out"=w627:errorcluster, "Queue Ref Out"=w623:refnum<queue>)  [unwired: 8 in]
                n249 = call "Enqueue Display Element.vi"("error in (no error)"=w627, "Display Console Data"=w624, "Display Console Message"=Display_Console_Message."Update Time", "Message Queue"=w623) -> ("error out"=w620:errorcluster)  [unwired: 6 in, 1 out]
                n250 = call "Controller Queue Reference Handler.vi"("Error In"=w620, "Reference Action"=Reference_Action."Get") -> ("Error Out"=w618:errorcluster, "Queue Ref Out"=w617:refnum<queue>)  [unwired: 8 in]
                n251 = To Variant(anything=Timer_Actions."Check Time" ("TimerAction")) -> (Variant=w614:variant)
                n252 = call "Enqueue Controller Element.vi"("error in (no error)"=w618, "Controller Queue Data"=w614, "Controller Queue Message"=Controller_Queue_Message."Check Time", "Message Queue"=w617) -> ("error out"=w613:errorcluster)  [unwired: 6 in, 1 out]
              }
              frame True {
                n253 = call "Check Direction.vi"("error in (no error)"=w634, "Controller Data Cluster"=w631) -> ("error out"=w633:errorcluster, "Direction"=w632:T4)  [unwired: 8 in]
                n254 = call "Request.vi"("error in (no error)"=w633, "Controller Data Cluster"=w631) -> ("error out"=w635:errorcluster, "Request?"=w636:bool)  [unwired: 8 in]
                n255 = Bundle By Name(cluster=w631, "Current Direction"=w632) -> (w630:T1)
                n256 = case shown="True" w636 {
                  tunnel: w635 -> [w640 w650]
                  tunnel: [w638 w646] -> w637
                  frame False {
                    n257 = call "Controller Queue Reference Handler.vi"("Error In"=w640, "Reference Action"=Reference_Action."Get") -> ("Error Out"=w639:errorcluster, "Queue Ref Out"=w643:refnum<queue>)  [unwired: 8 in]
                    n258 = call "Enqueue Controller Element.vi"("error in (no error)"=w639, "Controller Queue Message"=Controller_Queue_Message."No Request Remaining", "Message Queue"=w643) -> ("error out"=w638:errorcluster)  [unwired: 7 in, 1 out]
                  }
                  frame True {
                    w653 = T12 {"User Event Enum"=enum."Disable Open/Close Controlls", "UI Data Cluster"={"Floor Selection"=[], "Elevator Call Up"=[], "Elevator Call Down"=[], "Door Buttons"={"Open"=FALSE, "Close"=FALSE}, "Emergency"=FALSE}}  # User Event Cluster
                    n259 = call "User Event Reference Handler.vi"("Reference Action"=Reference_Action."Get", "Error In"=w650) -> ("Error Out"=w654:errorcluster, "User Event Refnum Out"=w651:refnum<user-event>)  [unwired: 7 in, 1 out]
                    n260 = To Variant(anything=w653) -> (Variant=w652:variant)
                    n261 = Generate User Event(user event=w651, event data cluster=w652, error in=w654) -> (error out=w647:errorcluster)  [unwired: 1 in, 1 out]
                    n262 = call "Controller Queue Reference Handler.vi"("Error In"=w647, "Reference Action"=Reference_Action."Get") -> ("Error Out"=w648:errorcluster, "Queue Ref Out"=w645:refnum<queue>)  [unwired: 8 in]
                    n263 = call "Enqueue Controller Element.vi"("error in (no error)"=w648, "Controller Queue Message"=Controller_Queue_Message."Start and Move", "Message Queue"=w645) -> ("error out"=w646:errorcluster)  [unwired: 7 in, 1 out]
                  }
                }
              }
            }
          }
        }
      }
      frame "Start Exit" {
        w662 = T12 {"User Event Enum"=enum."Controller Loop Closed", "UI Data Cluster"={"Floor Selection"=[], "Elevator Call Up"=[], "Elevator Call Down"=[], "Door Buttons"={"Open"=FALSE, "Close"=FALSE}, "Emergency"=FALSE}}  # Update Controlls Cluster
        n264 = call "Controller Queue Reference Handler.vi"("Error In"=w659, "Reference Action"=Reference_Action."Get") -> ("Error Out"=w658:errorcluster, "Queue Ref Out"=w656:refnum<queue>)  [unwired: 8 in]
        n265 = Flush Queue(queue=w656, error in (no error)=w658) -> (error out=w657:errorcluster)  [unwired: 2 out]
        n266 = call "User Event Reference Handler.vi"("Reference Action"=Reference_Action."Get", "Error In"=w657) -> ("Error Out"=w674:errorcluster, "User Event Refnum Out"=w675:refnum<user-event>)  [unwired: 7 in, 1 out]
        n267 = To Variant(anything=w662) -> (Variant=w661:variant)
        n268 = Generate User Event(user event=w675, event data cluster=w661, error in=w674) -> (error out=w671:errorcluster)  [unwired: 1 in, 1 out]
        n269 = call "Display Queue Reference Handler.vi"("Error In"=w671, "Reference Action"=Reference_Action."Get") -> ("Error Out"=w670:errorcluster, "Queue Ref Out"=w672:refnum<queue>)  [unwired: 8 in]
        n270 = call "Enqueue Display Element.vi"("error in (no error)"=w670, "Display Console Message"=Display_Console_Message."Exit", "Message Queue"=w672) -> ("error out"=w667:errorcluster)  [unwired: 7 in, 1 out]
        n271 = call "Sensor User Event Reference Handler.vi"("Reference Action"=Reference_Action."Get", "Error In"=w667) -> ("Error Out"=w668:errorcluster, "User Event Refnum Out"=w664:refnum<user-event>)  [unwired: 7 in, 1 out]
        n272 = Generate User Event(user event=w664, event data cluster=variant ("event data"), error in=w668) -> (error out=w666:errorcluster)  [unwired: 1 in, 1 out]
      }
      frame "Close Door" {
        w682 = T9 {"Timing"=0.0, "Elevator Location"=0, "Elevator Direction"={"Up"=FALSE, "Down"=FALSE}, "Door Open"=FALSE, "Emergency"=FALSE}  # Display Console Data Cluster
        w688 = T12 {"User Event Enum"=enum."Disable Open Door Controll", "UI Data Cluster"={"Floor Selection"=[], "Elevator Call Up"=[], "Elevator Call Down"=[], "Door Buttons"={"Open"=FALSE, "Close"=FALSE}, "Emergency"=FALSE}}  # User Event Cluster
        n273 = Bundle By Name(cluster=w693, "Timed Action"=Timed_Action."Close Door") -> (w692:T1)
        n274 = call "Controller Queue Reference Handler.vi"("Error In"=w697, "Reference Action"=Reference_Action."Get") -> ("Error Out"=w700:errorcluster, "Queue Ref Out"=w699:refnum<queue>)  [unwired: 8 in]
        n275 = To Variant(anything=Timer_Actions."Reset" ("TimerAction")) -> (Variant=w695:variant)
        n276 = call "Enqueue Controller Element.vi"("error in (no error)"=w700, "Controller Queue Data"=w695, "Controller Queue Message"=Controller_Queue_Message."Check Time", "Message Queue"=w699) -> ("error out"=w679:errorcluster)  [unwired: 6 in, 1 out]
        n277 = call "User Event Reference Handler.vi"("Reference Action"=Reference_Action."Get", "Error In"=w679) -> ("Error Out"=w691:errorcluster, "User Event Refnum Out"=w690:refnum<user-event>)  [unwired: 7 in, 1 out]
        n278 = To Variant(anything=w688) -> (Variant=w687:variant)
        n279 = Generate User Event(user event=w690, event data cluster=w687, error in=w691) -> (error out=w680:errorcluster)  [unwired: 1 in, 1 out]
        n280 = To Variant(anything=w682) -> (Variant=w681:variant)
        n281 = call "Display Queue Reference Handler.vi"("Error In"=w680, "Reference Action"=Reference_Action."Get") -> ("Error Out"=w683:errorcluster, "Queue Ref Out"=w686:refnum<queue>)  [unwired: 8 in]
        n282 = call "Enqueue Display Element.vi"("error in (no error)"=w683, "Display Console Data"=w681, "Display Console Message"=Display_Console_Message."Update", "Message Queue"=w686) -> ("error out"=w678:errorcluster)  [unwired: 6 in, 1 out]
      }
    }
  }
  "Error Out" <- w2
